vi "SRV_List System Configs.vi"(0 "Config Dir":path, 11 "error in (no error)":errorcluster) -> (4 "Config Dir dup":path, 8 "System Config Names":string[](array[string]), 15 "error out":errorcluster)   [LabVIEW 2014]
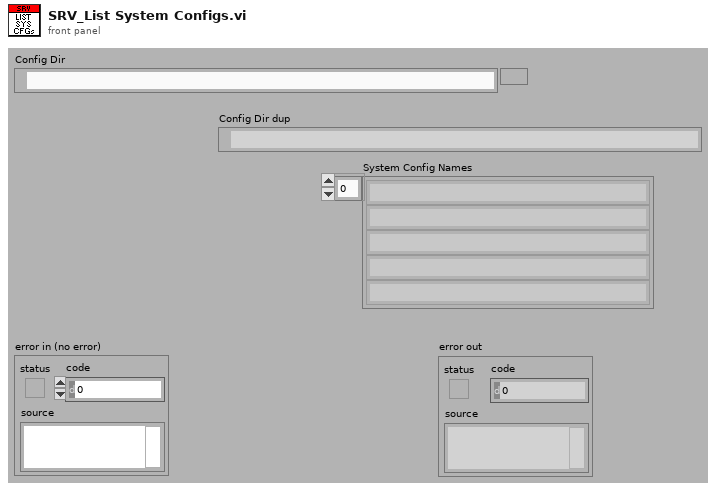
[diagram p1: front panel]
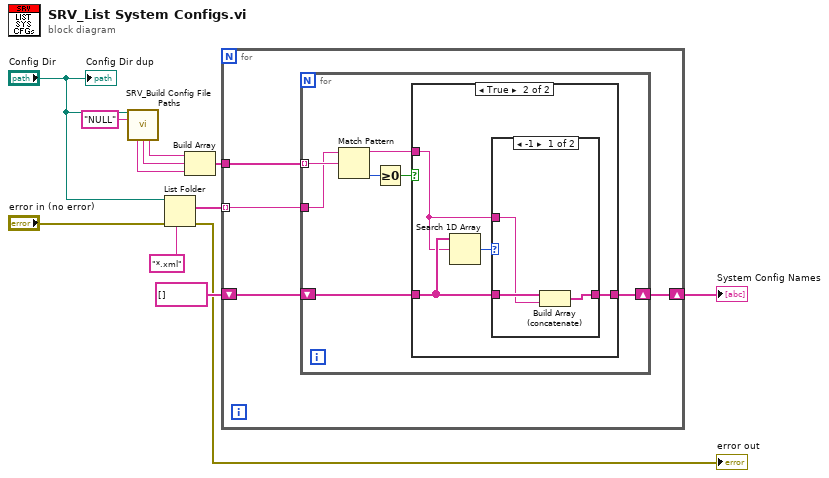
[diagram p0: block diagram]
diagram:
  n1 = call "SRV_Build Config File Paths.vi"("Config Dir"="Config Dir", "Sys Config Name"="NULL") -> ("SensorsConfig regexp"=w8:string, "MotorsConfig regexp"=w7:string, "SystemConfig regexp"=w6:string)  [unwired: 8 in, 3 out]
  n2 = List Folder(path="Config Dir", pattern="*.xml", error in="error in (no error)") -> (filenames=w5:string[], error out=→"error out":errorcluster)  [unwired: 1 in, 2 out]
  n3 = Build Array(w6, w7, w8) -> (w9:string[])
  n4 = for {
    tunnel: w5 -> [w15] mode=indexing
    tunnel: w9 -> [w16]
    shift-right: [w13] -> w11
    shift-left: string[] [] -> [w14]
    n5 = for {
      tunnel: w16 -> [w23] mode=indexing
      tunnel: w15 -> [w22]
      shift-right: [w17] -> w13
      shift-left: w14 -> [w18]
      n6 = Match Pattern(string=w22, regular expression=w23) -> (before substring=w20:string, offset past match=w21:i32)  [unwired: 1 in, 2 out]
      n7 = Greater Or Equal To 0?(x=w21) -> (x >= 0?=w19:bool)
      n8 = case shown="True" w19 {
        tunnel: w20 -> [_ w25]
        tunnel: w18 -> [w24 w27]
        tunnel: [w24 w26] -> w17
        frame False {
        }
        frame True {
          n9 = Search 1D Array(1D array=w27, element=w25) -> (index of element=w28:i32)  [unwired: 1 in]
          n10 = case shown="-1" w28 {
            tunnel: w27 -> [w31 w32]
            tunnel: [w30 w32] -> w26
            tunnel: w25 -> [w29 _]
            frame -1 {
              n11 = Build Array (concatenate)(w31, w29) -> (w30:string[])
            }
            frame Default {
            }
          }
        }
      }
    }
  }
  "System Config Names" <- w11
  "Config Dir dup" <- "Config Dir"
